vi "Motion@WaitMotor__Parameter.vi"(1 "ParamterIn":string) -> (0 "ParamterOut":string)   [LabVIEW 2019]
panel:
  in  "Message":string(combo)
  in  "TimeOut":string(combo)
  in  "MotorSelect":string(combo)
  in  "Confirm":bool
  # "Motion@WaitMotor $Motor(,$Timeout=XX,[[$label]]$Message)"
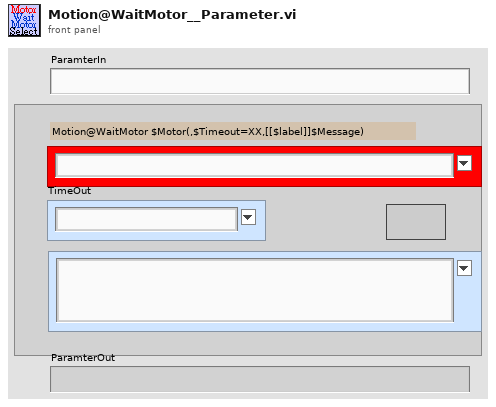
[diagram p1: front panel]
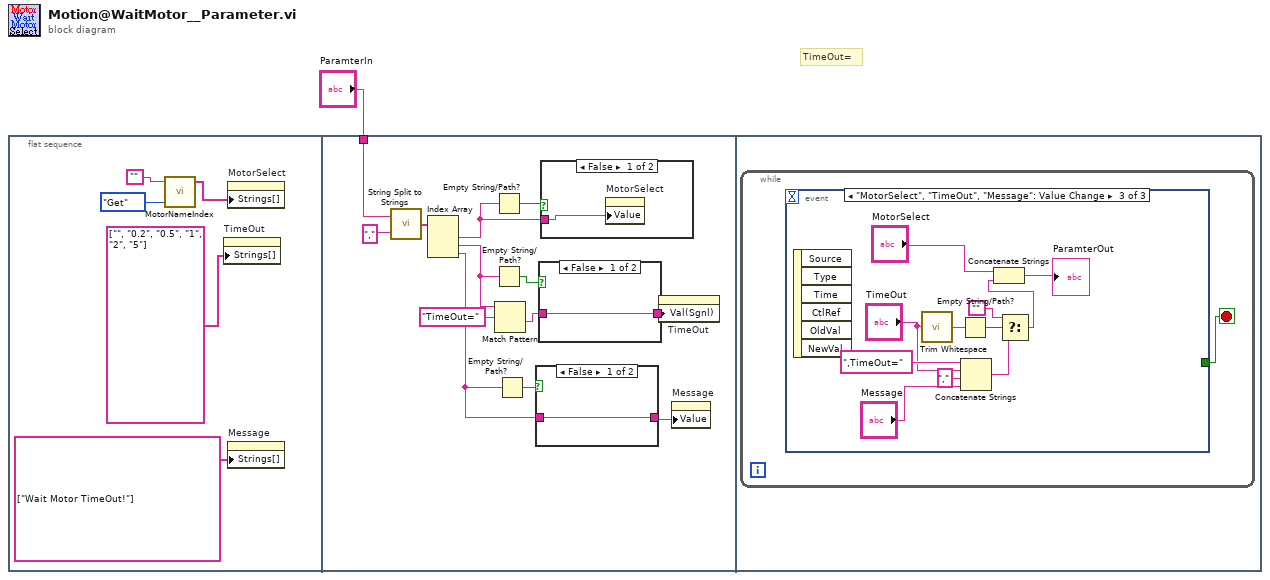
[diagram p0: block diagram]
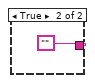
[diagram p2: hidden frame]
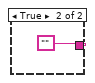
[diagram p3: hidden frame]
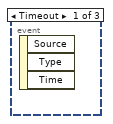
[diagram p5: hidden frame]
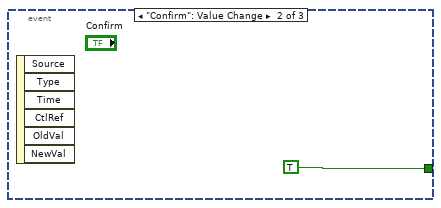
[diagram p6: hidden frame]
diagram:
  # "TimeOut="
  n1 = flat-sequence {
    tunnel: "ParamterIn" -> [w17]
    frame #0 {
      n2 = call "MotorNameIndex.vi"("OP"=enum16{"Get", "Update", "Init"}."Get", "MotorName"="") -> ("MotorList"=w3:string[])  [unwired: 1 in, 2 out]
      n3 = property on="TimeOut" class="CmbBox"("Strings[]"=string[] ["", "0.2", "0.5", "1", "2", "5"] ("Strings []")) -> ()  [unwired: 2 in, 2 out]
      n4 = property on="MotorSelect" class="CmbBox"("Strings[]"=w3) -> ()  [unwired: 2 in, 2 out]
      n5 = property on="Message" class="CmbBox"("Strings[]"=string[] ["Wait Motor TimeOut!"] ("Strings []")) -> ()  [unwired: 2 in, 2 out]
    }
    frame #1 {
      n6 = call "String Split to Strings.vi"("search string/char (-)"=",", "String"=w17) -> ("Array"=w19:string[])
      n7 = Index Array(array=w19) -> (element #1=w15:string, element #2=w12:string, element #3=w8:string)  [unwired: 3 in]
      n8 = Empty String/Path?(string/path=w15) -> (empty?=w16:bool)
      n9 = Empty String/Path?(string/path=w12) -> (empty?=w14:bool)
      n10 = Match Pattern(string=w12, regular expression="TimeOut=") -> (after substring=w10:string)  [unwired: 1 in, 3 out]
      n11 = Empty String/Path?(string/path=w8) -> (empty?=w9:bool)
      n12 = case shown="False" w9 {
        tunnel: [w20 ""] -> w7
        tunnel: w8 -> [w20 _]
        frame False {
        }
        frame True {
        }
      }
      n13 = case shown="False" w14 {
        tunnel: [w22 ""] -> w13
        tunnel: w10 -> [w22 _]
        frame False {
        }
        frame True {
        }
      }
      n14 = case shown="False" w16 {
        tunnel: w15 -> [w24 _]
        frame False {
          n15 = property on="MotorSelect" class="CmbBox"("Value"=w24) -> ()  [unwired: 2 in, 2 out]
        }
        frame True {
        }
      }
      n16 = property on="TimeOut" class="CmbBox"("Val(Sgnl)"=w13) -> ()  [unwired: 2 in, 2 out]
      n17 = property on="Message" class="CmbBox"("Value"=w7) -> ()  [unwired: 2 in, 2 out]
    }
    frame #2 {
      n18 = while {
        stop <- w25 stop-if-true
        n19 = event shown="[2] \"MotorSelect\", \"TimeOut\", \"Message\": Value Change" {
          selector: _ -> [_ _ _]
          dyn-events: _ -> [_ _ _]
          timeout: _ -> [_ _ _]
          tunnel: [_ TRUE _] -> w25
          event Timeout {
            n20 = event-data() -> ()  [unwired: 1 in, 3 out]
          }
          event "Confirm": Value Change {
            n21 = event-data() -> ()  [unwired: 1 in, 6 out]
          }
          event "MotorSelect", "TimeOut", "Message": Value Change {
            n22 = event-data() -> ()  [unwired: 1 in, 6 out]
            n23 = call <vilib>:"Trim Whitespace.vi"("string"="TimeOut") -> ("trimmed string"=w31:string)  [unwired: 1 in]
            n24 = Empty String/Path?(string/path=w31) -> (empty?=w32:bool)
            n25 = Concatenate Strings(",TimeOut=" ("string"), "TimeOut", "," ("string"), "Message") -> (w34:string)
            n26 = Select(t="", s=w32, f=w34) -> (s? t:f=w29:string)
            n27 = Concatenate Strings("MotorSelect", w29) -> (→"ParamterOut":string)
          }
        }
      }
    }
  }
